vi "Set Cache Out of Date.vi"(11 "Graphic.lvclass":refnum<class "Graphic.lvclass">) -> (3 "Graphic.lvclass out":refnum<class "Graphic.lvclass">)   [LabVIEW 2018, in "Graphic.lvclass"]
doc: "Use this VI to mark the cache as invalid so that the class renders the graphic on next draw."
uses:
  Graphic.lvclass
  Graphic.lvclass/Graphic.ctl
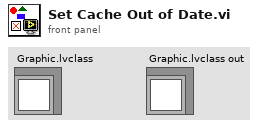
[diagram p1: front panel]
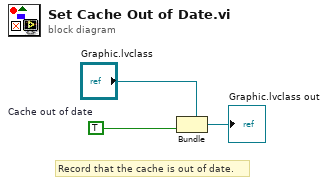
[diagram p0: block diagram]
diagram:
  w1 = TRUE  # Cache out of date
  # "Record that the cache is out of date."
  n1 = Bundle(cluster="Graphic.lvclass", w1) -> (→"Graphic.lvclass out":refnum<class "Graphic.lvclass">)  [unwired: 1 out]
